vi "SetPropertiesValue.vi"(7 "Index":i32, 8 "error in (no error)":errorcluster, 10 "Variant":variant, 11 "JSON":string="{}") -> (0 "error out":errorcluster, 3 "<JSON>":string)   [LabVIEW 2017]
uses:
  <vilib>/JDP Science/JSONtext/JSONtext.lvlib
  3b661bee-1ee3-4b8c-b689-ee013f4a4403.vi
  9bd81b63-e180-47be-93aa-f6adeb3ef81a.vi
  15420834-eb6d-4624-9ea5-33a89ea5d8cd.vi
  <vilib>/Utility/Data Type/NI_Data Type.lvlib
  4dc68120-58c9-423c-9dd9-51e81b41a9cb.vi
  8968c855-941f-43c1-9567-9c01a34c92a1.vi
  a839fead-af43-4b6a-bfde-fef6da7a8869.vi
  66e2e543-9bae-4e56-a7b9-a603e5daffc5.vi
  872ecbff-d206-417d-8adb-6f0dfc49c4ca.vi
  8375a3dd-6031-4de2-9220-f4c506173f19.vi
  f6127b87-8433-45e3-a086-e215588d9822.vi
  23ceb002-abd5-48ea-864e-537e4f58b202.vi
  5301696e-f7fe-4ea3-a706-bcc876a8d0b0.vi
  ae9afca5-8f48-42b1-a84a-ef1c047755b5.vi
  de05bbdd-603a-4cad-8eab-e5299d04d8f8.vi
  31410703-653f-4077-acd0-9f2558e53ad4.vi
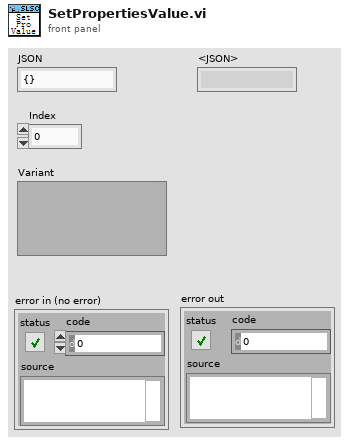
[diagram p1: front panel]
types:
  T1 = typedef "NI_Data Type.lvlib/Data Type.ctl" = enum8{"Invalid Type", "Void", "I8", "I16", "I32", "I64", "U8", "U16", "U32", "U64", "Single Float", "Double Float", "Extended Float", "Single Complex", "Double Complex", "Extended Complex", "Enum U8", "Enum U16", "Enum U32", "Enum U64", "Single Float With Unit", "Double Float With Unit", "Extended Float With Unit", "Single Complex with Unit", "Double Complex with Unit", "Extended Complex with Unit", "Boolean", "String", "Path", "Picture", "Tag", "Array", "Cluster", "Variant", "LV Variant", "Waveform", "Timestamp", "Digital Waveform", "Digital Data", "ExpressData", "Refnum", "External Data", "VI", "Poly VI", "LabVIEW Class Instance", "Fixed Point"}
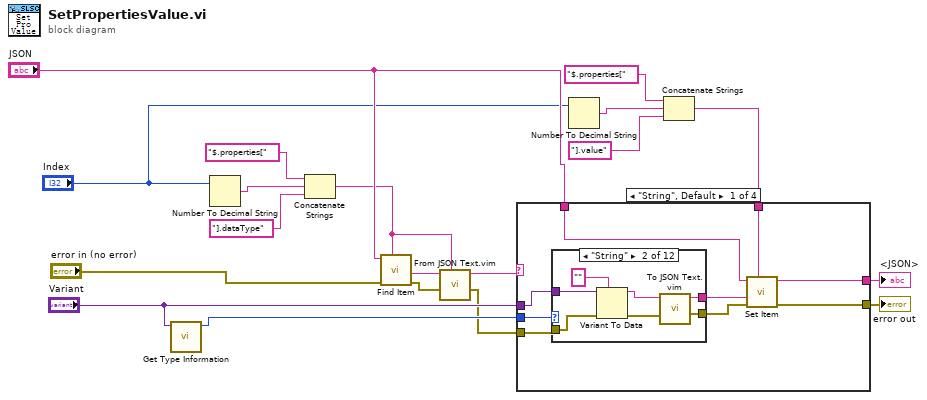
[diagram p0: block diagram]
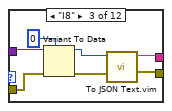
[diagram p3: hidden frame]
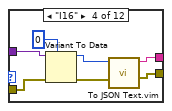
[diagram p4: hidden frame]
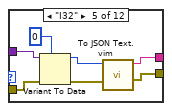
[diagram p5: hidden frame]
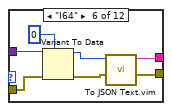
[diagram p6: hidden frame]
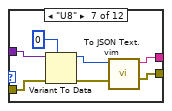
[diagram p7: hidden frame]
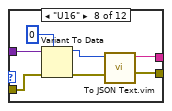
[diagram p8: hidden frame]
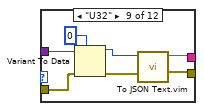
[diagram p9: hidden frame]
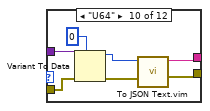
[diagram p10: hidden frame]
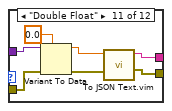
[diagram p11: hidden frame]
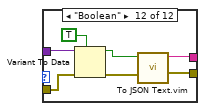
[diagram p12: hidden frame]
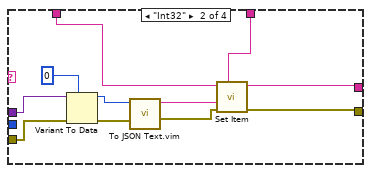
[diagram p13: hidden frame]
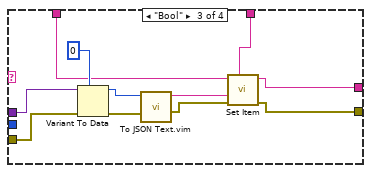
[diagram p14: hidden frame]
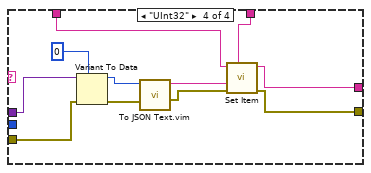
[diagram p15: hidden frame]
diagram:
  n1 = call <vilib>:"Get Type Information.vi"("Variant"="Variant") -> ("Type"=w5:T1)  [unwired: 6 in, 4 out]
  n2 = Number To Decimal String(number="Index") -> (decimal integer string=w8:string)  [unwired: 1 in]
  n3 = Concatenate Strings("$.properties[" ("format string"), w8, "].dataType") -> (w11:string)
  n4 = call <vilib>:"Find Item.vi"("$Path or Item Name"=w11, "error in (no error)"="error in (no error)", "JSON"="JSON") -> ("error out"=w3:errorcluster, "<JSON>"=w10:string)  [unwired: 5 in, 2 out]
  n5 = call "From JSON Text.vim"("Data Type and Default Value"=w11, "error in (no error)"=w3, "JSON"=w10) -> ("error out"=w2:errorcluster, "Data out"=w12:string)  [unwired: 7 in]
  n6 = Number To Decimal String(number="Index") -> (decimal integer string=w14:string)  [unwired: 1 in]
  n7 = Concatenate Strings("$.properties[" ("format string"), w14, "].value") -> (w17:string)
  n8 = case shown="\"String\", Default" w12 {
    tunnel: "Variant" -> [w28 w113 w128 w139]
    tunnel: "JSON" -> [w26 w114 w124 w135]
    tunnel: w17 -> [w25 w111 w123 w134]
    tunnel: [w24 w112 w122 w133] -> w18
    tunnel: w5 -> [w23 _ _ _]
    tunnel: w2 -> [w22 w110 w121 w132]
    tunnel: [w20 w107 w118 w129] -> w1
    frame "String", Default {
      n9 = case shown="\"String\"" w23 {
        tunnel: w28 -> [_ w36 w42 w49 w56 w63 w70 w77 w84 w91 w98 w104]
        tunnel: [_ w33 w40 w48 w54 w62 w68 w75 w82 w89 w96 w103] -> w27
        tunnel: w22 -> [w29 w32 w39 w46 w53 w60 w67 w74 w81 w88 w95 w102]
        tunnel: [w29 w30 w37 w44 w51 w58 w65 w72 w79 w86 w93 w100] -> w21
        frame "Invalid Type", Default {
        }
        frame "String" {
          n10 = Variant To Data(error in=w32, type="", Variant=w36) -> (data=w34:string, error out=w31:errorcluster)
          n11 = call "To JSON Text.vim"("error in (no error)"=w31, "Anything"=w34) -> ("error out"=w30:errorcluster, "<JSON>"=w33:string)  [unwired: 8 in]
        }
        frame "I8" {
          n12 = Variant To Data(error in=w39, type=i8 0, Variant=w42) -> (data=w43:i8, error out=w38:errorcluster)
          n13 = call "To JSON Text.vim"("error in (no error)"=w38, "Anything"=w43) -> ("error out"=w37:errorcluster, "<JSON>"=w40:string)  [unwired: 8 in]
        }
        frame "I16" {
          n14 = Variant To Data(error in=w46, type=i16 0, Variant=w49) -> (data=w50:i16, error out=w45:errorcluster)
          n15 = call "To JSON Text.vim"("error in (no error)"=w45, "Anything"=w50) -> ("error out"=w44:errorcluster, "<JSON>"=w48:string)  [unwired: 8 in]
        }
        frame "I32" {
          n16 = Variant To Data(error in=w53, type=0, Variant=w56) -> (data=w57:i32, error out=w52:errorcluster)
          n17 = call "To JSON Text.vim"("error in (no error)"=w52, "Anything"=w57) -> ("error out"=w51:errorcluster, "<JSON>"=w54:string)  [unwired: 8 in]
        }
        frame "I64" {
          n18 = Variant To Data(error in=w60, type=i64 0, Variant=w63) -> (data=w64:i64, error out=w59:errorcluster)
          n19 = call "To JSON Text.vim"("error in (no error)"=w59, "Anything"=w64) -> ("error out"=w58:errorcluster, "<JSON>"=w62:string)  [unwired: 8 in]
        }
        frame "U8" {
          n20 = Variant To Data(error in=w67, type=u8 0, Variant=w70) -> (data=w71:u8, error out=w66:errorcluster)
          n21 = call "To JSON Text.vim"("error in (no error)"=w66, "Anything"=w71) -> ("error out"=w65:errorcluster, "<JSON>"=w68:string)  [unwired: 8 in]
        }
        frame "U16" {
          n22 = Variant To Data(error in=w74, type=u16 0, Variant=w77) -> (data=w78:u16, error out=w73:errorcluster)
          n23 = call "To JSON Text.vim"("error in (no error)"=w73, "Anything"=w78) -> ("error out"=w72:errorcluster, "<JSON>"=w75:string)  [unwired: 8 in]
        }
        frame "U32" {
          n24 = Variant To Data(error in=w81, type=u32 0, Variant=w84) -> (data=w85:u32, error out=w80:errorcluster)
          n25 = call "To JSON Text.vim"("error in (no error)"=w80, "Anything"=w85) -> ("error out"=w79:errorcluster, "<JSON>"=w82:string)  [unwired: 8 in]
        }
        frame "U64" {
          n26 = Variant To Data(error in=w88, type=u64 0, Variant=w91) -> (data=w92:u64, error out=w87:errorcluster)
          n27 = call "To JSON Text.vim"("error in (no error)"=w87, "Anything"=w92) -> ("error out"=w86:errorcluster, "<JSON>"=w89:string)  [unwired: 8 in]
        }
        frame "Double Float" {
          n28 = Variant To Data(error in=w95, type=0.0, Variant=w98) -> (data=w99:dbl, error out=w94:errorcluster)
          n29 = call "To JSON Text.vim"("error in (no error)"=w94, "Anything"=w99) -> ("error out"=w93:errorcluster, "<JSON>"=w96:string)  [unwired: 8 in]
        }
        frame "Boolean" {
          n30 = Variant To Data(error in=w102, type=TRUE, Variant=w104) -> (data=w106:bool, error out=w101:errorcluster)
          n31 = call "To JSON Text.vim"("error in (no error)"=w101, "Anything"=w106) -> ("error out"=w100:errorcluster, "<JSON>"=w103:string)  [unwired: 8 in]
        }
      }
      n32 = call <vilib>:"Set Item.vi"("$Path or Item Name"=w25, "error in (no error)"=w21, "JSON to Insert"=w27, "JSON"=w26) -> ("error out"=w20:errorcluster, "<JSON>"=w24:string)  [unwired: 4 in, 1 out]
    }
    frame "Int32" {
      n33 = Variant To Data(error in=w110, type=0, Variant=w113) -> (data=w116:i32, error out=w109:errorcluster)
      n34 = call "To JSON Text.vim"("error in (no error)"=w109, "Anything"=w116) -> ("error out"=w108:errorcluster, "<JSON>"=w115:string)  [unwired: 8 in]
      n35 = call <vilib>:"Set Item.vi"("$Path or Item Name"=w111, "error in (no error)"=w108, "JSON to Insert"=w115, "JSON"=w114) -> ("error out"=w107:errorcluster, "<JSON>"=w112:string)  [unwired: 4 in, 1 out]
    }
    frame "Bool" {
      n36 = Variant To Data(error in=w121, type=u16 0, Variant=w128) -> (data=w126:u16, error out=w120:errorcluster)
      n37 = call "To JSON Text.vim"("error in (no error)"=w120, "Anything"=w126) -> ("error out"=w119:errorcluster, "<JSON>"=w125:string)  [unwired: 8 in]
      n38 = call <vilib>:"Set Item.vi"("$Path or Item Name"=w123, "error in (no error)"=w119, "JSON to Insert"=w125, "JSON"=w124) -> ("error out"=w118:errorcluster, "<JSON>"=w122:string)  [unwired: 4 in, 1 out]
    }
    frame "UInt32" {
      n39 = Variant To Data(error in=w132, type=u32 0, Variant=w139) -> (data=w137:u32, error out=w131:errorcluster)
      n40 = call "To JSON Text.vim"("error in (no error)"=w131, "Anything"=w137) -> ("error out"=w130:errorcluster, "<JSON>"=w136:string)  [unwired: 8 in]
      n41 = call <vilib>:"Set Item.vi"("$Path or Item Name"=w134, "error in (no error)"=w130, "JSON to Insert"=w136, "JSON"=w135) -> ("error out"=w129:errorcluster, "<JSON>"=w133:string)  [unwired: 4 in, 1 out]
    }
  }
  "<JSON>" <- w18
  "error out" <- w1
